vi "Data2.get.vi"(8 "error in (no error)":errorcluster, 11 "midi-file-event.midi in":refnum<class "midi-file-event.midi.lvclass">) -> (0 "error out":errorcluster, 2 "Data2":u8, 3 "midi-file-event.midi out":refnum<class "midi-file-event.midi.lvclass">)   [LabVIEW 2020, in "midi-file-event.midi.lvclass"]
uses:
  midi-file-event.midi.lvclass
  midi-file-event.midi.lvclass/midi-file-event.midi.ctl
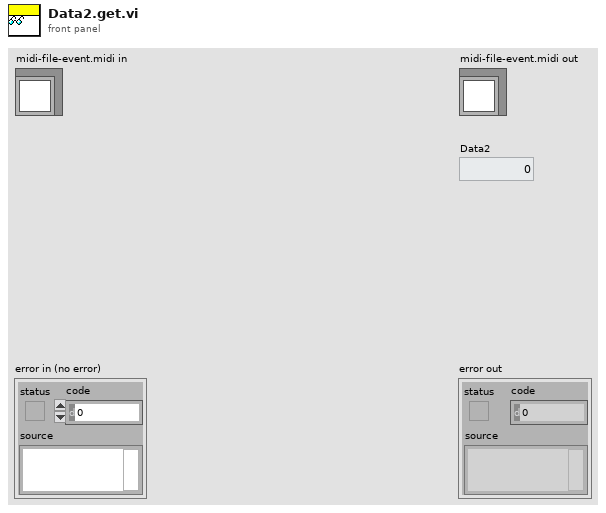
[diagram p1: front panel]
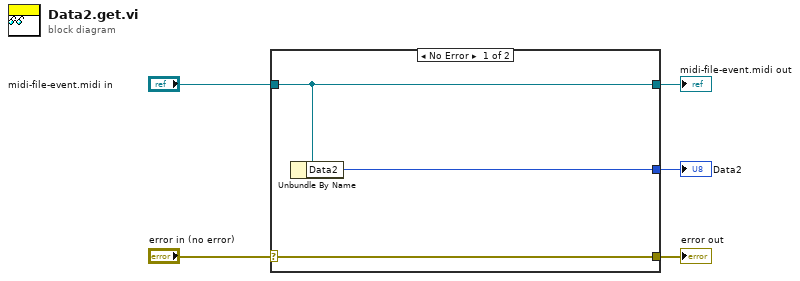
[diagram p0: block diagram]
diagram:
  n1 = case shown="No Error" "error in (no error)" {
    selector: "error in (no error)" -> [w8 w9]
    tunnel: [w8 w9] -> w4
    tunnel: [w7 w10] -> w2
    tunnel: "midi-file-event.midi in" -> [w7 w10]
    tunnel: [w6 _] -> w1
    frame No Error {
      n2 = Unbundle By Name(w7) -> ("Data2"=w6:u8)
    }
    frame Error {
    }
  }
  "error out" <- w4
  "midi-file-event.midi out" <- w2
  "Data2" <- w1
